vi "Read Stop .vi"(8 "error in (no error)":errorcluster, 11 "TTLController in":refnum<class "TTLController.lvclass">) -> (0 "error out":errorcluster, 2 "Trigger":T1, 3 "TTLController out":refnum<class "TTLController.lvclass">)   [LabVIEW 2020, in "TTLController.lvclass"]
uses:
  TTLController.lvclass
  Trigger.ctl
  TTLController.lvclass/TTLController.ctl
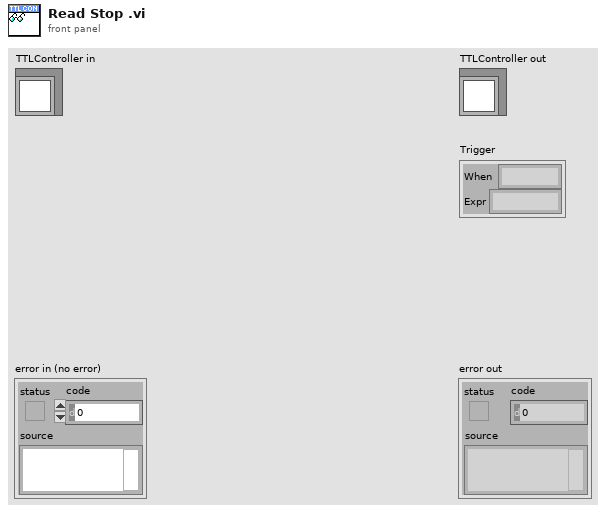
[diagram p1: front panel]
types:
  T1 = typedef "TTLController.lvclass/Trigger.ctl" = cluster{"When":string, "Expr":string}
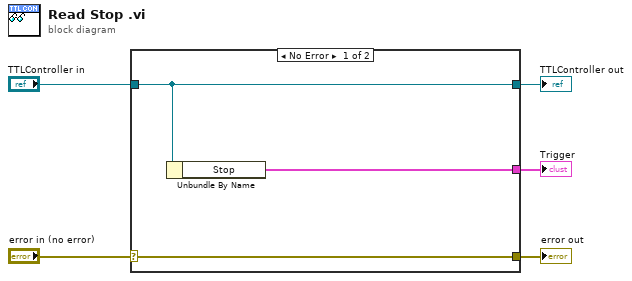
[diagram p0: block diagram]
diagram:
  n1 = case shown="No Error" "error in (no error)" {
    selector: "error in (no error)" -> [w8 w9]
    tunnel: [w8 w9] -> w4
    tunnel: [w7 w10] -> w2
    tunnel: "TTLController in" -> [w7 w10]
    tunnel: [w6 _] -> w1
    frame No Error {
      n2 = Unbundle By Name(w7) -> ("Stop"=w6:T1)
    }
    frame Error {
    }
  }
  "error out" <- w4
  "TTLController out" <- w2
  "Trigger" <- w1
